vi "Stop Core.vi"(10 "final error code":i32, 11 "Measurement Setup in":refnum<class "Measurement Setup.lvclass">) -> (3 "Measurement Setup out":refnum<class "Measurement Setup.lvclass">)   [LabVIEW 2015, in "Measurement Setup Controller.lvlib" / "Measurement Setup.lvclass"]
uses:
  Measurement Setup.lvclass
  <vilib>/ActorFramework/Message Enqueuer/Message Enqueuer.lvclass/Message Enqueuer.ctl
  <vilib>/ActorFramework/Message Enqueuer/Enqueue.vi
  <vilib>/ActorFramework/Message Priority Queue/Priority Enqueue.vi
  <userlib>/Common Components/Controller/Controller.lvclass
  <vilib>/ActorFramework/Stop Msg/Stop Msg.lvclass
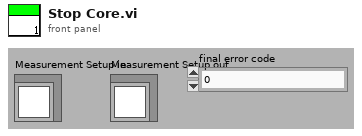
[diagram p1: front panel]
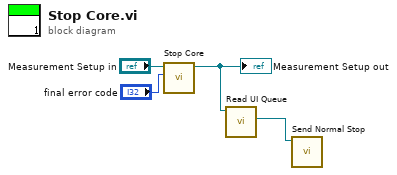
[diagram p0: block diagram]
diagram:
  n1 = call-parent "Stop Core.vi"("final error code"="final error code", "Controller in"="Measurement Setup in") -> ("Controller out"=w2:refnum<class "Measurement Setup.lvclass">)  [unwired: 9 in]
  "Measurement Setup out" <- w2
  n2 = call <userlib>:"Read UI Queue.vi"("UI Controller in"=w2) -> ("UI Queue"=w1:refnum<class "Message Enqueuer.lvclass">)  [unwired: 8 in, 2 out]
  n3 = call <vilib>:"Send Normal Stop.vi"("Message Enqueuer"=w1) -> ()  [unwired: 10 in, 1 out]
